vi "Parse Table HTML.vi"(11 "array of devices":T1) -> (3 "String":string)   [LabVIEW 2016]
uses:
  Array Device Info.ctl
  Device Info.ctl
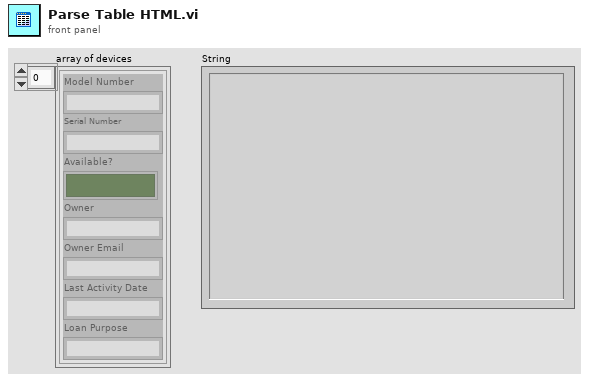
[diagram p1: front panel]
types:
  T1 = typedef "Array Device Info.ctl" = T2[]
  T2 = typedef "Device Info.ctl" = cluster{"Model Number":string, "Serial Number":string, "Available?":bool, "Owner":string, "Owner Email":string, "Last Activity Date":string, "Loan Purpose":string}
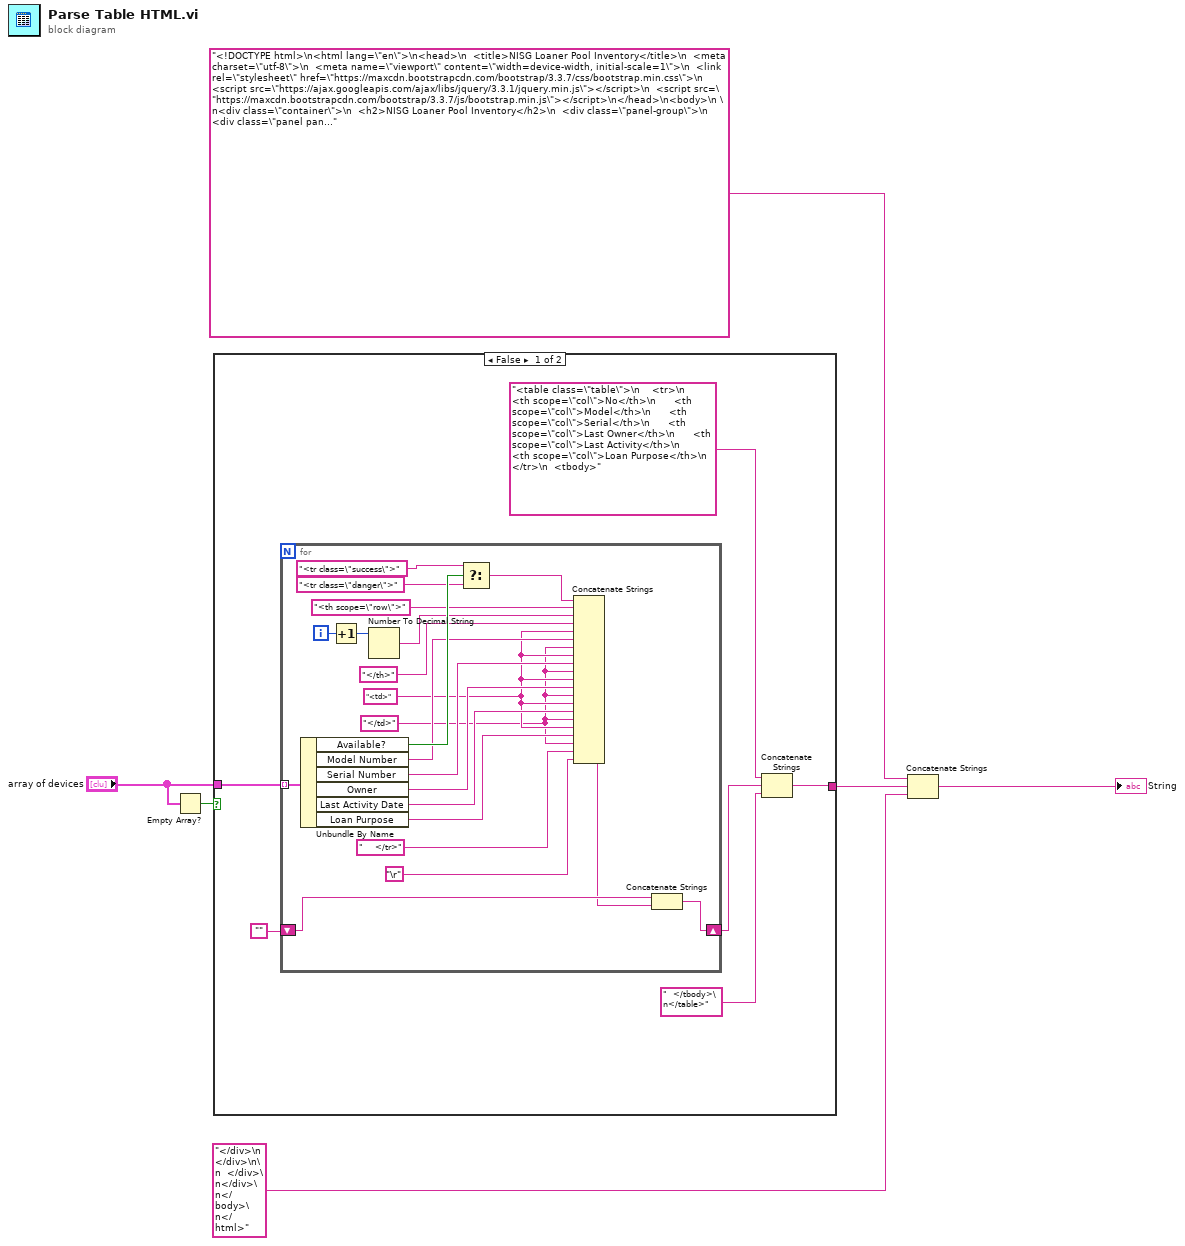
[diagram p0: block diagram]
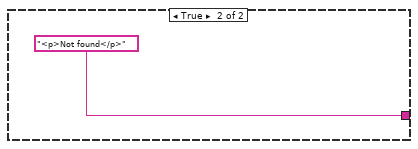
[diagram p2: hidden frame]
diagram:
  n1 = Empty Array?(array="array of devices") -> (empty?=w1:bool)
  n2 = case shown="False" w1 {
    tunnel: "array of devices" -> [w12 _]
    tunnel: [w7 "<p>Not found</p>"] -> w4
    frame False {
      n3 = for {
        tunnel: w12 -> [w34] mode=indexing
        shift-right: [w13] -> w9
        shift-left: "" -> [w15]
        i -> [w30]
        w18 = "</td>"
        w20 = "<td>"
        n4 = Unbundle By Name(w34) -> ("Available?"=w33:bool, "Model Number"=w24:string, "Serial Number"=w23:string, "Owner"=w22:string, "Last Activity Date"=w21:string, "Loan Purpose"=w19:string)
        n5 = Increment(x=w30) -> (x+1=w29:i32)
        n6 = Number To Decimal String(number=w29) -> (decimal integer string=w26:string)  [unwired: 1 in]
        n7 = Select(t="<tr class=\"success\">", s=w33, f="<tr class=\"danger\">") -> (s? t:f=w28:string)
        n8 = Concatenate Strings(w28, "<th scope=\"row\">", w26, "</th>", w20, w24, w18, w20, w23, w18, w20, w22, w18, w20, w21, w18, w20, w19, w18, "    </tr>", "\r") -> (w14:string)
        n9 = Concatenate Strings(w15, w14) -> (w13:string)
      }
      n10 = Concatenate Strings("<table class=\"table\">\n    <tr>\n      <th scope=\"col\">No</th>\n      <th scope=\"col\">Model</th>\n      <th scope=\"col\">Serial</th>\n      <th scope=\"col\">Last Owner</th>\n      <th scope=\"col\">Last Activity</th>\n      <th scope=\"col\">Loan Purpose</th>\n    </tr>\n  <tbody>", w9, "  </tbody>\n</table>") -> (w7:string)
    }
    frame True {
    }
  }
  n11 = Concatenate Strings("<!DOCTYPE html>\n<html lang=\"en\">\n<head>\n  <title>NISG Loaner Pool Inventory</title>\n  <meta charset=\"utf-8\">\n  <meta name=\"viewport\" content=\"width=device-width, initial-scale=1\">\n  <link rel=\"stylesheet\" href=\"https://maxcdn.bootstrapcdn.com/bootstrap/3.3.7/css/bootstrap.min.css\">\n  <script src=\"https://ajax.googleapis.com/ajax/libs/jquery/3.3.1/jquery.min.js\"></script>\n  <script src=\"https://maxcdn.bootstrapcdn.com/bootstrap/3.3.7/js/bootstrap.min.js\"></script>\n</head>\n<body>\n \n<div class=\"container\">\n  <h2>NISG Loaner Pool Inventory</h2>\n  <div class=\"panel-group\">\n    <div class=\"panel panel-primary\">\n      <div class=\"panel-heading\"><h3><strong>Search results</strong><h3>\n\t  </div>\n      <div class=\"panel-body\">\n        \n        \n      ", w4, "</div>\n    </div>\n\n  </div>\n</div>\n</body>\n</html>") -> (→"String":string)
